vi "LMS Adaptive Filtering (V1.00).vi"(0 "Time Data":refnum<class "GSwFormDSP.lvclass">, 5 "error in (no error)":errorcluster, 7 "Application Name":string="AdvSigProc", 9 "State Queue":T3[](array[typedef])=["SC >>> Initialize"]) -> (19 "error out":errorcluster)   [LabVIEW 2020, in "AdvSigProc.lvclass"]
uses:
  AdvSigProc.lvclass
  API/Generic Utilities_class/utils/GenUtil State List.ctl
  API/GSwFormDSP_class/GSwFormDSP.lvclass
  protected/LMS Input Parameters.ctl
  <vilib>/Utility/sysdir.llb/System Directory Type.ctl
  API/GSwFormDSP_class/functions/Attribute Options.ctl
  SPWB_class/Controls/Analysis Type.ctl
  C:/Users/fcharett/docsWork/coding/20openSourceSPWB/API/Generic Utilities_class/Generic Utilities.lvclass
  <vilib>/Platform/browser.llb/Open URL in Default Browser (path).vi
  <vilib>/addons/_AddQ/G#Object/G#Object.lvclass
  API/Generic Utilities_class/Generic Utilities.lvclass
  File IO/TDMS_class/TDMS.lvclass
  SPWB_class/SPWB.lvclass
panel:
  in  "Task":T1(tab)
  in  "Noisy Signal (X +n)":u16(ring) items=["MidSunvisor Array Center", "Voice Signal"]
  in  "Reference Signal (X)":u16(ring) items=["MidSunvisor Array Center", "Voice Signal"]
  in  "Input Parameters":T2={"Type"=enum."Normalized LMS", "Filter Class"=enum."Noise Cancelling (BGN Ref)", "Filter Length"=256, "µ Parameters"={"Type"=enum."User Input", "step size"=1.0}, "Iterations"={"Current"=1, "Maximum"=1000}} {"µ Parameters"."step size" scale=1e-08..1.0}
  in  "LMS Start/Stop":bool
  in  "TDP LMS Results":bool
  out "Filter Coefs":dbl[](graph)
  in  "Filtered Signals":waveform(dbl)[](graph)
  out "Iterations.Current":i32
  in  "Open TDMS":bool
  in  "Time Signal":waveform(dbl)[](graph)
  out "Current File":path
  in  "AppData Folder":bool
  out "State History":string[](array[string])
  out "State Index":i32
  out "Exec Time":dbl
  in  "TimeOut":i32=-1 caption="msec"
  in  "Exit":bool
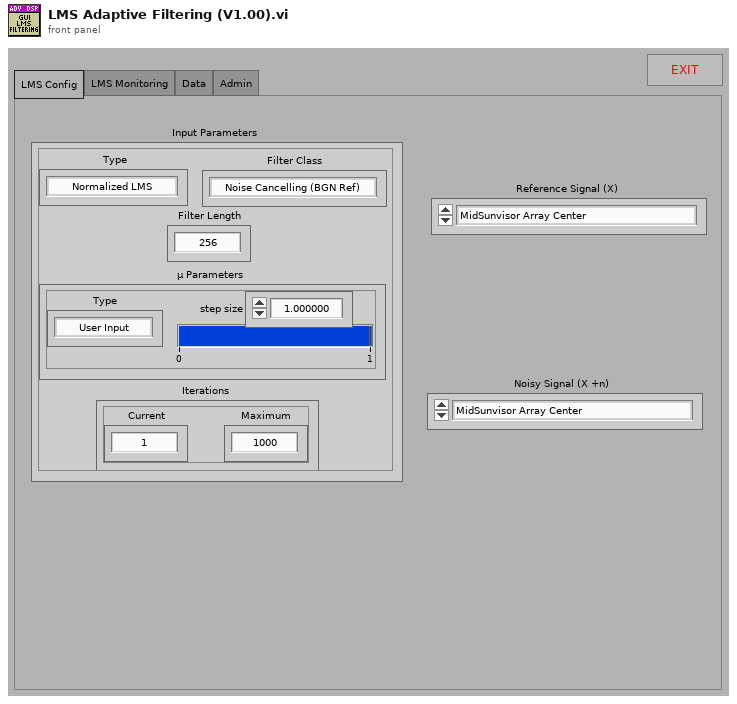
[diagram p1: front panel]
types:
  T1 = enum32{"LMS Config", "LMS Monitoring", "Data", "Admin"}
  T2 = typedef "AdvSigProc.lvclass/LMS Input Parameters.ctl" = cluster{"Type":enum16{"Normalized LMS", "LMS", "FIR Sign LMS", "FIR Fast Block LMS", "RLS", "QR - RLS"}, "Filter Class":enum16{"Noise Cancelling (BGN Ref)", "Noise Cancelling (Speech Ref)"}, "Filter Length":i32, "µ Parameters":cluster{"Type":enum16{"User Input", "Auto µ"}, "step size":dbl}, "Iterations":cluster{"Current":i32, "Maximum":i32}}
  T3 = typedef "Generic Utilities.lvclass/GenUtil State List.ctl" = string
  T4 = typedef "SPWB.lvclass/Analysis Type.ctl" = enum16{"Time Data Processing", "FFT Analysis", "Time Frequency Analysis", "Transfer Functions"}
  T5 = typedef "GSwFormDSP.lvclass/Attribute Options.ctl" = enum16{"Append to Attribute using \"( )\"", "Replace Attribute Value"}
  T6 = enum32{"Invalid", "Standard", "Closed", "Hidden", "Minimized", "Maximized"}
  T7 = typedef "System Directory Type.ctl" = i32
  T8 = cluster{"Window Name Index":string, "wForm Ref":refnum<class "GSwFormDSP.lvclass">}[]
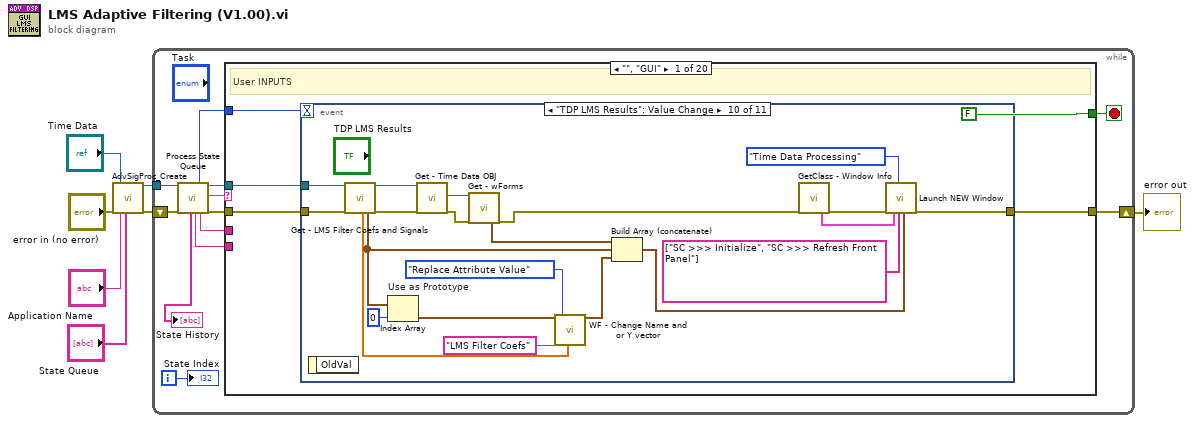
[diagram p0: block diagram]
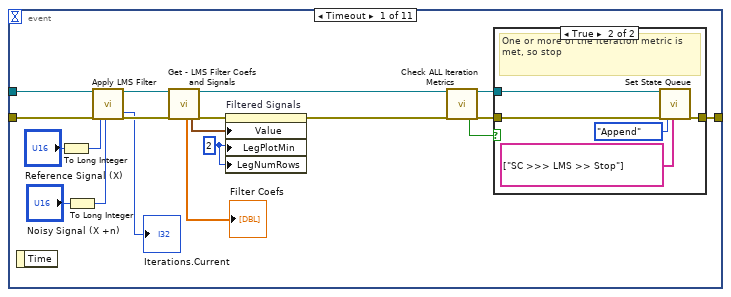
[diagram p2: hidden frame]
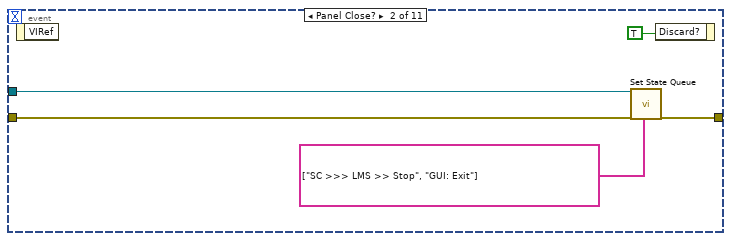
[diagram p4: hidden frame]
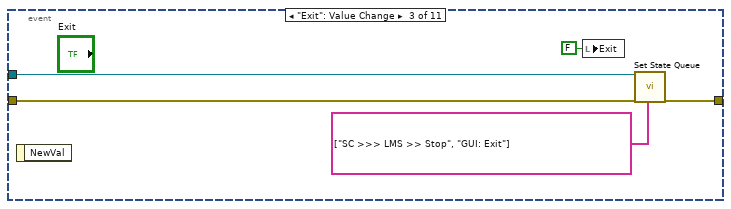
[diagram p5: hidden frame]
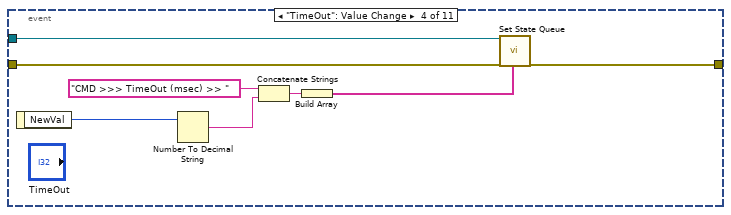
[diagram p6: hidden frame]
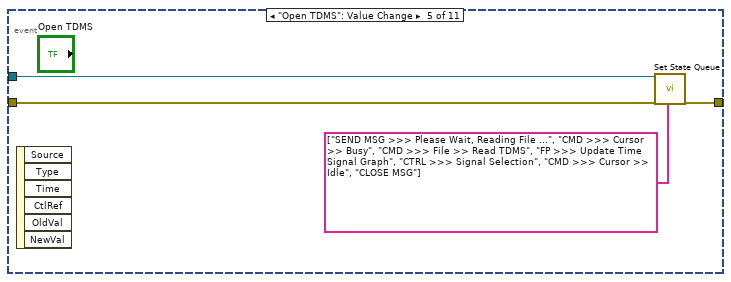
[diagram p7: hidden frame]
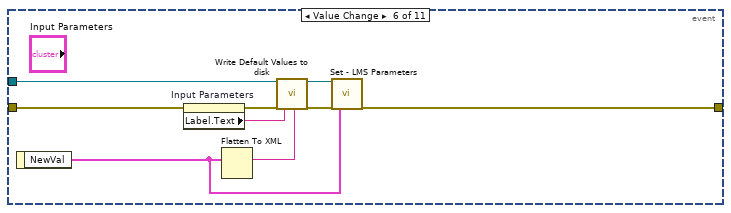
[diagram p8: hidden frame]
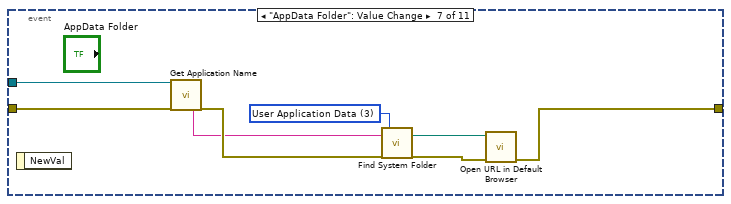
[diagram p9: hidden frame]
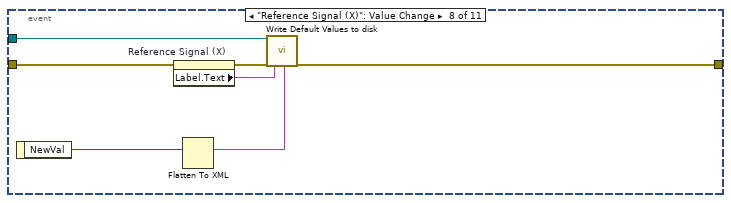
[diagram p10: hidden frame]
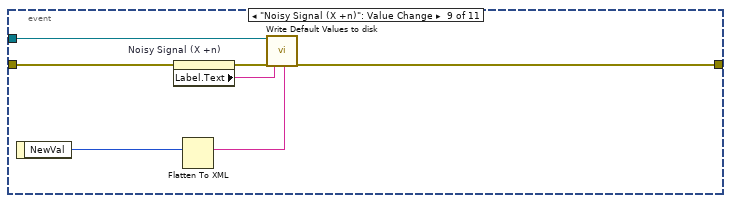
[diagram p11: hidden frame]
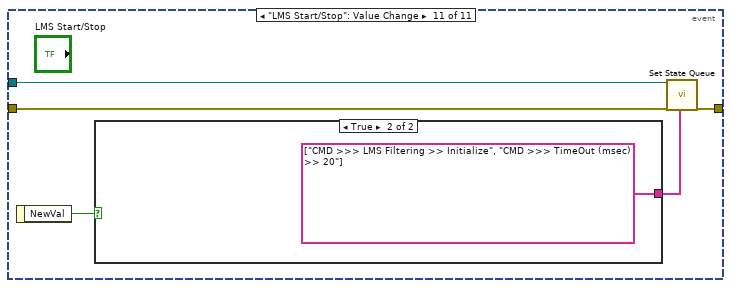
[diagram p12: hidden frame]
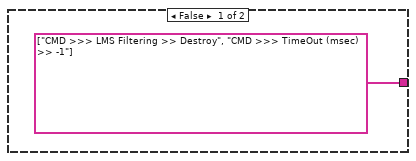
[diagram p13: hidden frame]
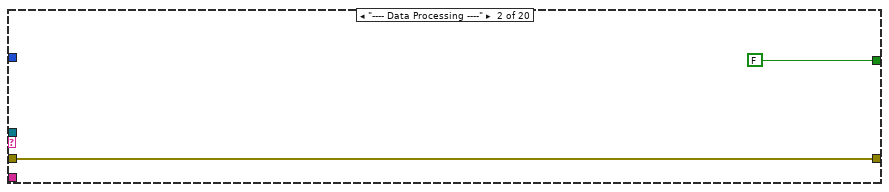
[diagram p14: hidden frame]
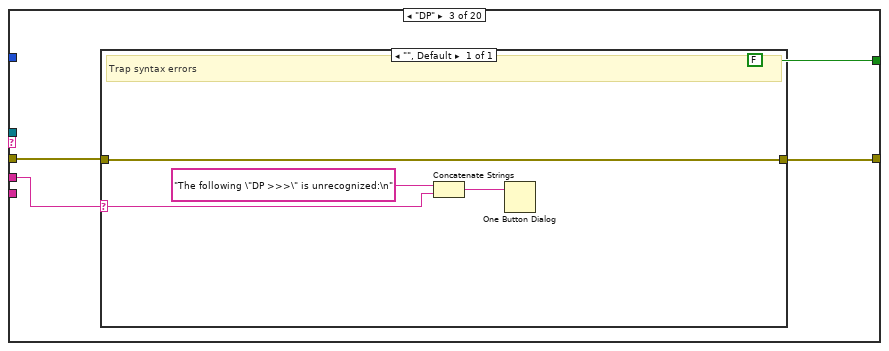
[diagram p15: hidden frame]
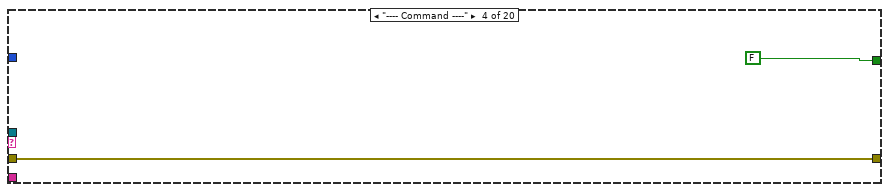
[diagram p16: hidden frame]
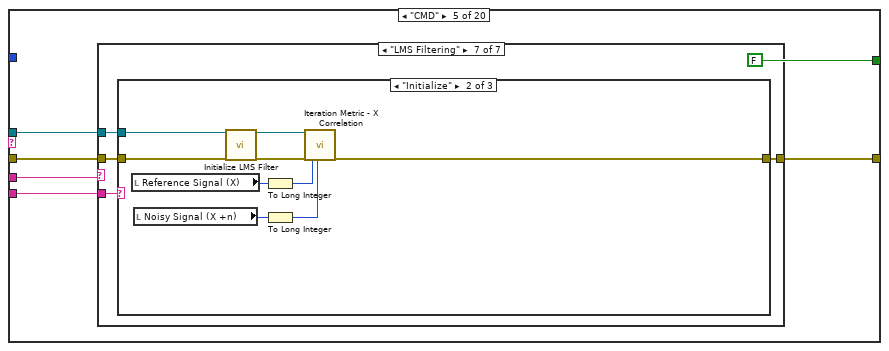
[diagram p17: hidden frame]
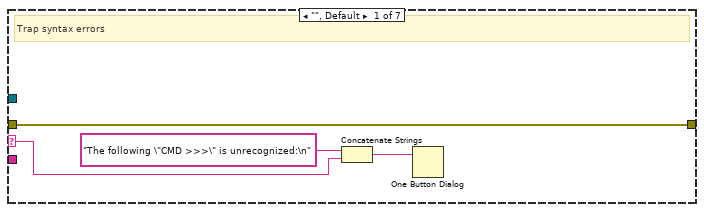
[diagram p18: hidden frame]
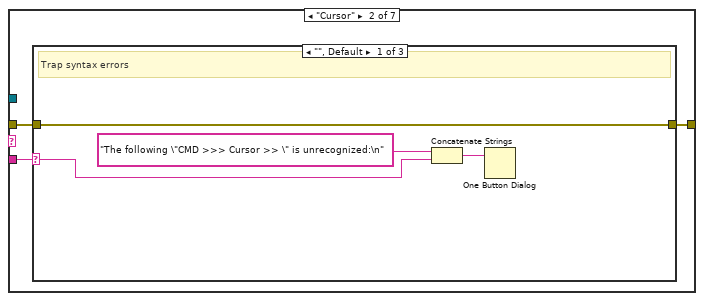
[diagram p19: hidden frame]
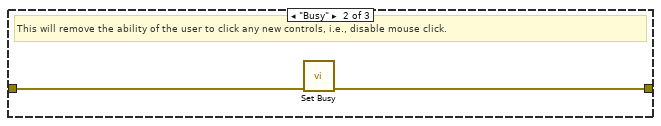
[diagram p20: hidden frame]
diagram:
  n1 = call "AdvSigProc_Create.vi"("error in (no error)"="error in (no error)", "Time Data"="Time Data", "Application Name"="Application Name", "State Queue"="State Queue") -> ("reference out"=w7:refnum<class "AdvSigProc.lvclass">, "error out"=w6:errorcluster)  [unwired: 14 in]
  n2 = while {
    shift-right: [w11] -> w2
    shift-left: w6 -> [w16]
    tunnel: w7 -> [w17]
    i -> [w18]
    stop <- w19 stop-if-true
    n3 = call "Process State Queue.vi"("reference in"=w17, "error in (no error)"=w16) -> ("State History"=→"State History":string[], "Additional Options"=w8:string, "Timeout"=w15:i32, "State Option"=w10:string, "reference out"=w14:refnum<class "AdvSigProc.lvclass">, "Current State"=w13:string, "error out"=w12:errorcluster)  [unwired: 10 in, 1 out]
    n4 = case shown="\"\", \"GUI\"" w13 {
      selector: w13 -> [_ _ _ _ _ _ _ _ _ _ _ _ _ _ _ _ w485 _ _ _]
      tunnel: w14 -> [w22 _ _ _ w143 _ w238 _ w257 w371 _ w413 w439 w474 w478 _ _ _ _ w495]
      tunnel: [FALSE FALSE FALSE FALSE FALSE FALSE FALSE FALSE FALSE FALSE FALSE FALSE TRUE FALSE FALSE FALSE FALSE FALSE FALSE TRUE] -> w19
      tunnel: w15 -> [w23 _ _ _ _ _ _ _ _ _ _ _ _ _ _ _ _ _ _ _]
      tunnel: w10 -> [_ _ w135 _ w147 _ w234 _ w258 w368 _ _ _ w471 _ _ _ _ _ _]
      tunnel: w12 -> [w21 w131 w134 w141 w145 w230 w237 w252 w255 w370 w399 w411 w436 w473 w479 w481 w483 w488 w491 w494]
      tunnel: [w20 w131 w133 w141 w146 w230 w236 w252 w256 w369 w399 w401 w435 w472 w477 w481 w483 errorcluster {"status"=FALSE, "code"=0, "source"=""} ("error out") w491 w493] -> w11
      tunnel: w8 -> [_ _ _ _ w144 _ w232 _ w254 _ _ _ _ _ _ _ _ _ _ _]
      frame "", "GUI" {
        # "User INPUTS"
        n5 = event shown="[9] \"TDP LMS Results\": Value Change" {
          selector: _ -> [_ _ _ _ _ _ _ _ _ _ _]
          dyn-events: _ -> [_ _ _ _ _ _ _ _ _ _ _]
          timeout: w23 -> [_ _ _ _ _ _ _ _ _ _ _]
          tunnel: w22 -> [w42 w53 w58 w63 w70 w80 w87 w92 w99 w121 w127]
          tunnel: w21 -> [w43 w52 w56 w62 w69 w77 w86 w93 w100 w120 w126]
          tunnel: [w30 w51 w57 w61 w71 w73 w81 w89 w96 w104 w125] -> w20
          event Timeout {
            w33 = u32 2
            n6 = event-data() -> ()  [unwired: 1 in, 1 out]
            n7 = To Long Integer(number="Reference Signal (X)") -> (32bit integer=w38:i32)
            n8 = To Long Integer(number="Noisy Signal (X +n)") -> (32bit integer=w39:i32)
            n9 = call "Apply LMS Filter.vi"("reference in"=w42, "error in (no error)"=w43, "Reference Signal"=w38, "Response Signal"=w39) -> ("Iterations.Current"=→"Iterations.Current":i32, "reference out"=w37:refnum<class "AdvSigProc.lvclass">, "error out"=w36:errorcluster)  [unwired: 13 in]
            n10 = call "Get - LMS Filter Coefs and Signals.vi"("reference in"=w37, "error in (no error)"=w36) -> ("Filter Coefs"=→"Filter Coefs":dbl[], "LMS Filtered Signals"=w34:waveform(dbl)[], "reference out"=w29:refnum<class "AdvSigProc.lvclass">, "error out"=w35:errorcluster)  [unwired: 14 in]
            n11 = property on="Filtered Signals" class="WFGraph (strict)"(error in=w35, "Value"=w34, "LegPlotMin"=w33, "LegNumRows"=w33) -> (error out=w27:errorcluster)  [unwired: 1 in, 1 out]
            n12 = call "Check ALL Iteration Metrics.vi"("reference in"=w29, "error in (no error)"=w27) -> ("Stop Iteration"=w25:bool, "reference out"=w28:refnum<class "AdvSigProc.lvclass">, "error out"=w26:errorcluster)  [unwired: 15 in]
            n13 = case shown="True" w25 {
              tunnel: w26 -> [w44 w48]
              tunnel: w28 -> [_ w47]
              tunnel: [w44 w46] -> w30
              frame False {
                # "Go to the next iteration!"
              }
              frame True {
                # "One or more of the iteration metric is met, so stop"
                n14 = call "Set State Queue.vi"("reference in"=w47, "error in (no error)"=w48, "State Queue Options"=enum16{"Replace", "Append", "Prepend"}."Append", "State Queue"=string[] ["SC >>> LMS >> Stop"]) -> ("error out"=w46:errorcluster)  [unwired: 14 in, 1 out]
              }
            }
          }
          event Panel Close? {
            n15 = event-data() -> ()  [unwired: 1 in, 1 out]
            n16 = call "Set State Queue.vi"("reference in"=w53, "error in (no error)"=w52, "State Queue"=string[] ["SC >>> LMS >> Stop", "GUI: Exit"]) -> ("error out"=w51:errorcluster)  [unwired: 15 in, 1 out]
            n17 = event-data("Discard?"=TRUE) -> ()  [unwired: 1 in, 1 out]
          }
          event "Exit": Value Change {
            n18 = event-data() -> ()  [unwired: 1 in, 1 out]
            n19 = local write "Exit"(FALSE ("Exit")) -> ()
            n20 = call "Set State Queue.vi"("reference in"=w58, "error in (no error)"=w56, "State Queue"=string[] ["SC >>> LMS >> Stop", "GUI: Exit"]) -> ("error out"=w57:errorcluster)  [unwired: 15 in, 1 out]
          }
          event "TimeOut": Value Change {
            n21 = event-data() -> ("NewVal"=w60:i32)  [unwired: 1 in]
            n22 = Number To Decimal String(number=w60) -> (decimal integer string=w65:string)  [unwired: 1 in]
            n23 = Concatenate Strings("CMD >>> TimeOut (msec) >> " ("String"), w65) -> (w66:string)
            n24 = Build Array(w66) -> (w67:string[])
            n25 = call "Set State Queue.vi"("reference in"=w63, "error in (no error)"=w62, "State Queue"=w67) -> ("error out"=w61:errorcluster)  [unwired: 15 in, 1 out]
          }
          event "Open TDMS": Value Change {
            n26 = event-data() -> ()  [unwired: 1 in, 6 out]
            n27 = call "Set State Queue.vi"("reference in"=w70, "error in (no error)"=w69, "State Queue"=string[] ["SEND MSG >>> Please Wait, Reading File ...", "CMD >>> Cursor >> Busy", "CMD >>> File >> Read TDMS", "FP >>> Update Time Signal Graph", "CTRL >>> Signal Selection", "CMD >>> Cursor >> Idle", "CLOSE MSG"]) -> ("error out"=w71:errorcluster)  [unwired: 15 in, 1 out]
          }
          event Value Change {
            n28 = event-data() -> ("NewVal"=w72:T2)  [unwired: 1 in]
            n29 = property on="Input Parameters" class="Clust (strict)"(error in=w77) -> (error out=w76:errorcluster, "Label.Text"=w79:string)  [unwired: 1 in, 1 out]
            n30 = Flatten To XML(6:w72) -> (2:w78:string)
            n31 = call-dynamic "Write Default Values to disk.vi"("reference in"=w80, "error in (no error)"=w76, "Control Label"=w79, "Value (XML String)"=w78) -> ("reference out"=w74:refnum<class "AdvSigProc.lvclass">, "error out"=w75:errorcluster)  [unwired: 14 in]
            n32 = call "Set - LMS Parameters.vi"("reference in"=w74, "error in (no error)"=w75, "Input Parameters"=w72) -> ("error out"=w73:errorcluster)  [unwired: 15 in, 1 out]
          }
          event "AppData Folder": Value Change {
            w88 = T7 3 items=["User Home"=0, "User Desktop"=1, "User Documents"=2, "User Application Data"=3, "User Preferences"=4, "User Temporary"=5, "Public Documents"=6, "Public Application Data"=7, "Public Preferences"=8, "Public Cache"=13, "System Core Libraries"=9, "System Installed Libraries"=10, "Application Files"=11, "Boot Volume Root"=12] ("system directory type")
            n33 = event-data() -> ()  [unwired: 1 in, 1 out]
            n34 = call "Get Application Name.vi"("reference in"=w87, "error in (no error)"=w86) -> ("Application Name"=w84:string, "error out"=w85:errorcluster)  [unwired: 15 in, 1 out]
            n35 = call "Find System Folder.vi"("Application Name"=w84, "error in (no error)"=w85, "system directory type"=w88) -> ("System Folder"=w83:path, "error out"=w82:errorcluster)  [unwired: 15 in]
            n36 = call-poly <vilib>:"Open URL in Default Browser.vi"("error in (no error)"=w82, "path"=w83) -> ("error out"=w81:errorcluster)  [unwired: 4 in, 1 out]
          }
          event "Reference Signal (X)": Value Change {
            n37 = event-data() -> ("NewVal"=w91:u16)  [unwired: 1 in]
            n38 = property on="Reference Signal (X)" class="Ring (strict)"(error in=w93) -> (error out=w94:errorcluster, "Label.Text"=w95:string)  [unwired: 1 in, 1 out]
            n39 = Flatten To XML(6:w91) -> (2:w90:string)
            n40 = call-dynamic "Write Default Values to disk.vi"("reference in"=w92, "error in (no error)"=w94, "Control Label"=w95, "Value (XML String)"=w90) -> ("error out"=w89:errorcluster)  [unwired: 14 in, 1 out]
          }
          event "Noisy Signal (X +n)": Value Change {
            n41 = event-data() -> ("NewVal"=w98:u16)  [unwired: 1 in]
            n42 = property on="Noisy Signal (X +n)" class="Ring (strict)"(error in=w100) -> (error out=w101:errorcluster, "Label.Text"=w102:string)  [unwired: 1 in, 1 out]
            n43 = Flatten To XML(6:w98) -> (2:w97:string)
            n44 = call-dynamic "Write Default Values to disk.vi"("reference in"=w99, "error in (no error)"=w101, "Control Label"=w102, "Value (XML String)"=w97) -> ("error out"=w96:errorcluster)  [unwired: 14 in, 1 out]
          }
          event "TDP LMS Results": Value Change {
            n45 = event-data() -> ()  [unwired: 1 in, 1 out]
            n46 = call "Get - LMS Filter Coefs and Signals.vi"("reference in"=w121, "error in (no error)"=w120) -> ("Filter Coefs"=w116:dbl[], "LMS Filtered Signals"=w111:waveform(dbl)[], "reference out"=w119:refnum<class "AdvSigProc.lvclass">, "error out"=w118:errorcluster)  [unwired: 14 in]
            n47 = Index Array "Use as Prototype"(array=w111, index=0) -> (element=w113:waveform(dbl))
            n48 = call "Get - Time Data OBJ.vi"("reference in"=w119, "error in (no error)"=w118) -> ("GSwFormDSP"=w123:refnum<class "GSwFormDSP.lvclass">, "error out"=w122:errorcluster)  [unwired: 14 in, 2 out]
            n49 = call-dynamic "Get - wForms.vi"("reference in"=w123, "error in (no error)"=w122) -> ("wForms"=w110:waveform(dbl)[], "error out"=w106:errorcluster)  [unwired: 14 in, 2 out]
            n50 = call "WF - Change Name and or Y vector.vi"("wForm IN"=w113, "Attribute Option"=Attribute_Options."Replace Attribute Value", "SigName Update"="LMS Filter Coefs", "New Y Data"=w116) -> ("wForm OUT"=w112:waveform(dbl))  [unwired: 14 in, 1 out]
            n51 = Build Array (concatenate)(w110, w111, w112) -> (w105:waveform(dbl)[])
            n52 = call "GetClass - Window Info.vi"("error in (no error)"=w106) -> ("Window Info"=w109:T8, "error out"=w108:errorcluster)  [unwired: 17 in]
            n53 = call "Launch NEW Window.vi"("error in (no error)"=w108, "Window Info"=w109, "Window Type"=Analysis_Type."Time Data Processing", "State Queue"=string[] ["SC >>> Initialize", "SC >>> Refresh Front Panel"], "wForms"=w105) -> ("error OUT"=w104:errorcluster)  [unwired: 14 in]
          }
          event "LMS Start/Stop": Value Change {
            n54 = event-data() -> ("NewVal"=w124:bool)  [unwired: 1 in]
            n55 = case shown="True" w124 {
              tunnel: [string[] ["CMD >>> LMS Filtering >> Destroy", "CMD >>> TimeOut (msec) >> -1"] ("State Queue") string[] ["CMD >>> LMS Filtering >> Initialize", "CMD >>> TimeOut (msec) >> 20"] ("State Queue")] -> w128
              frame False {
              }
              frame True {
              }
            }
            n56 = call "Set State Queue.vi"("reference in"=w127, "error in (no error)"=w126, "State Queue"=w128) -> ("error out"=w125:errorcluster)  [unwired: 15 in, 1 out]
          }
        }
      }
      frame "---- Data Processing ----" {
      }
      frame "DP" {
        n57 = case shown="\"\", Default" w135 {
          selector: w135 -> [w138]
          tunnel: [w137] -> w133
          tunnel: w134 -> [w137]
          frame "", Default {
            # "Trap syntax errors"
            n58 = Concatenate Strings("The following \"DP >>>\" is unrecognized:\n", w138) -> (w139:string)
            n59 = One Button Dialog(message=w139) -> ()  [unwired: 1 in, 1 out]
          }
        }
      }
      frame "---- Command ----" {
      }
      frame "CMD" {
        n60 = case shown="\"LMS Filtering\"" w147 {
          selector: w147 -> [w150 _ _ _ _ _ _]
          tunnel: [w149 w154 w166 w185 w187 w194 w212] -> w146
          tunnel: w145 -> [w149 w153 w165 w185 w188 w193 w211]
          tunnel: w144 -> [_ w155 w167 w182 w190 w195 w213]
          tunnel: w143 -> [_ _ w164 _ w189 w192 w210]
          frame "", Default {
            # "Trap syntax errors"
            n61 = Concatenate Strings("The following \"CMD >>>\" is unrecognized:\n", w150) -> (w151:string)
            n62 = One Button Dialog(message=w151) -> ()  [unwired: 1 in, 1 out]
          }
          frame "Cursor" {
            n63 = case shown="\"\", Default" w155 {
              selector: w155 -> [w157 _ _]
              tunnel: [w156 w160 w162] -> w154
              tunnel: w153 -> [w156 w161 w163]
              frame "", Default {
                # "Trap syntax errors"
                n64 = Concatenate Strings("The following \"CMD >>> Cursor >> \" is unrecognized:\n", w157) -> (w158:string)
                n65 = One Button Dialog(message=w158) -> ()  [unwired: 1 in, 1 out]
              }
              frame "Busy" {
                # "This will remove the ability of the user to click any new controls, i.e., disable mouse click."
                n66 = call <vilib>:"Set Busy.vi"("error in (no error)"=w161) -> ("error out"=w160:errorcluster)  [unwired: 9 in, 1 out]
              }
              frame "Idle" {
                # "Re-enables mouse click"
                n67 = call <vilib>:"Unset Busy.vi"("error in (no error)"=w163) -> ("error out"=w162:errorcluster)  [unwired: 10 in]
              }
            }
          }
          frame "Timer" {
            # "Can be use to time the execution or delays in processing or acquisition."
            n68 = case shown="\"\", Default" w167 {
              selector: w167 -> [w169 _ _]
              tunnel: [w168 w173 w178] -> w166
              tunnel: w165 -> [w168 w174 w179]
              tunnel: w164 -> [_ w175 w180]
              frame "", Default {
                # "Trap syntax errors"
                n69 = Concatenate Strings("The following \"CMD >>> Timer >> \" is unrecognized:\n", w169) -> (w170:string)
                n70 = One Button Dialog(message=w170) -> ()  [unwired: 1 in, 1 out]
              }
              frame "Start" {
                n71 = Get Date/Time In Seconds() -> (seconds since 1Jan1904=w172:timestamp)
                n72 = call "Set Timer Start.vi"("reference in"=w175, "error in (no error)"=w174, "Timer Start"=w172) -> ("error out"=w173:errorcluster)  [unwired: 15 in, 1 out]
              }
              frame "Stop" {
                n73 = call "Get Timer Start.vi"("reference in"=w180, "error in (no error)"=w179) -> ("Timer Start"=w177:timestamp, "error out"=w178:errorcluster)  [unwired: 15 in, 1 out]
                n74 = Get Date/Time In Seconds() -> (seconds since 1Jan1904=w181:timestamp)
                n75 = Subtract(x=w181, y=w177) -> (x-y=→"Exec Time":dbl)
              }
            }
          }
          frame "Wait (ms)" {
            # "Forces a time out"
            n76 = Decimal String To Number(string=w182, default (0L)=u32 0 ("default (0 I32)")) -> (number=w183:u32)  [unwired: 1 in, 1 out]
            n77 = Wait (ms)(milliseconds to wait=w183) -> ()  [unwired: 1 out]
          }
          frame "TimeOut (msec)" {
            # "Setup the default loop time out"
            n78 = Decimal String To Number(string=w190, default (0L)=0 ("default (0 I32)")) -> (number=w186:i32)  [unwired: 1 in, 1 out]
            n79 = call "Set State TimeOut.vi"("reference in"=w189, "error in (no error)"=w188, "TimeOut (msec)"=w186) -> ("error out"=w187:errorcluster)  [unwired: 15 in, 1 out]
            n80 = local write "TimeOut"(w186) -> ()
          }
          frame "File" {
            n81 = case shown="\"Read TDMS\"" w195 {
              selector: w195 -> [w197 _]
              tunnel: [w196 w200] -> w194
              tunnel: w193 -> [w196 w208]
              tunnel: w192 -> [_ w209]
              frame "", Default {
                n82 = Concatenate Strings("The following \"CMD >>> File >>\" is unrecognized:\n", w197) -> (w198:string)
                n83 = One Button Dialog(message=w198) -> ()  [unwired: 1 in, 1 out]
              }
              frame "Read TDMS" {
                n84 = call "Get Application Name.vi"("reference in"=w209, "error in (no error)"=w208) -> ("Application Name"=w203:string, "reference out"=w207:refnum<class "AdvSigProc.lvclass">, "error out"=w206:errorcluster)  [unwired: 15 in]
                n85 = call "Get - Time Data OBJ.vi"("reference in"=w207, "error in (no error)"=w206) -> ("GSwFormDSP"=w205:refnum<class "GSwFormDSP.lvclass">, "error out"=w204:errorcluster)  [unwired: 14 in, 2 out]
                n86 = call "GUI - TDMS (V2.00).vi"("Time Data IN"=w205, "error in (no error)"=w204, "Application Name"=w203, "State Queue"=string[] ["CMD: Prompt For READ Path", "CMD: Read File", "Quit"]) -> ("Loaded File"=→"Current File":path, "error out"=w200:errorcluster)  [unwired: 13 in, 1 out]
              }
            }
          }
          frame "LMS Filtering" {
            n87 = case shown="\"Initialize\"" w213 {
              selector: w213 -> [w215 _ _]
              tunnel: [w214 w218 w227] -> w212
              tunnel: w211 -> [w214 w225 w228]
              tunnel: w210 -> [_ w226 w229]
              frame "", Default {
                n88 = Concatenate Strings("The following \"CMD >>> LMS Filtering >>\" is unrecognized:\n", w215) -> (w216:string)
                n89 = One Button Dialog(message=w216) -> ()  [unwired: 1 in, 1 out]
              }
              frame "Initialize" {
                n90 = local read "Reference Signal (X)"() -> (w222:u16)
                n91 = local read "Noisy Signal (X +n)"() -> (w220:u16)
                n92 = call "Initialize LMS Filter.vi"("reference in"=w226, "error in (no error)"=w225) -> ("reference out"=w223:refnum<class "AdvSigProc.lvclass">, "error out"=w224:errorcluster)  [unwired: 16 in]
                n93 = To Long Integer(number=w222) -> (32bit integer=w221:i32)
                n94 = To Long Integer(number=w220) -> (32bit integer=w219:i32)
                n95 = call "Iteration Metric - X Correlation.vi"("reference in"=w223, "error in (no error)"=w224, "Reference Signal"=w221, "Response Signal"=w219) -> ("error out"=w218:errorcluster)  [unwired: 14 in, 1 out]
              }
              frame "Destroy" {
                n96 = call "Destroy LMS Filter.vi"("reference in"=w229, "error in (no error)"=w228) -> ("error out"=w227:errorcluster)  [unwired: 16 in, 1 out]
              }
            }
          }
        }
      }
      frame "---- Scripts ----" {
      }
      frame "SC" {
        n97 = case shown="\"LMS\"" w234 {
          selector: w234 -> [w241 _ _]
          tunnel: [string[] [] ("State Queue OUT") string[] ["GUI: Initialize Ref", "CTRL >>> Task Tab", "CTRL >>> LMS Parameters", "FP >>> Open"] ("State Queue OUT") w245] -> w235
          tunnel: w232 -> [_ _ w246]
          frame "False", Default {
            n98 = Concatenate Strings("The following \"Script\" is unrecognized:\n", w241) -> (w242:string)
            n99 = One Button Dialog(message=w242) -> ()  [unwired: 1 in, 1 out]
          }
          frame "Initialize" {
          }
          frame "LMS" {
            n100 = case shown="\"Stop\"" w246 {
              selector: w246 -> [w248 _]
              tunnel: [string[] [] ("State Queue OUT") string[] ["CMD >>> TimeOut (msec) >> -1", "CMD >>> LMS Filtering >> Destroy", "CTRL >>> LMS >> Stop"] ("State Queue OUT")] -> w245
              frame "", Default {
                n101 = Concatenate Strings("The following \"SC >>> LMS\" is unrecognized:\n", w248) -> (w249:string)
                n102 = One Button Dialog(message=w249) -> ()  [unwired: 1 in, 1 out]
              }
              frame "Stop" {
              }
            }
          }
        }
        n103 = call "Set State Queue.vi"("reference in"=w238, "error in (no error)"=w237, "State Queue Options"=enum16{"Replace", "Append", "Prepend"}."Prepend", "State Queue"=w235) -> ("error out"=w236:errorcluster)  [unwired: 14 in, 1 out]
      }
      frame "---- Front Panel Mgmt ----" {
      }
      frame "CTRL" {
        n104 = case shown="\"Signal Selection\"" w258 {
          selector: w258 -> [w262 _ _ _ _]
          tunnel: w257 -> [_ w267 w294 w330 _]
          tunnel: [w260 w265 w287 w305 w360] -> w256
          tunnel: w255 -> [w260 w266 w292 w329 w359]
          tunnel: w254 -> [_ _ _ _ w361]
          frame "unknown", Default {
            n105 = Concatenate Strings("The following control name is unrecognized:\n", w262) -> (w261:string)
            n106 = One Button Dialog(message=w261) -> ()  [unwired: 1 in, 1 out]
          }
          frame "Task Tab" {
            n107 = disable-structure shown="Enabled" {
              disable-tunnel: [w276 0] -> w268
              disable-tunnel: w267 -> [w274 _]
              disable-tunnel: w266 -> [w272 w284]
              disable-tunnel: [w269 w284] -> w264
              frame Disabled {
                n108 = property on="Task" class="TabCtl (strict)"(error in=w272) -> (error out=w273:errorcluster, "Label.Text"=w271:string, "Value"=w275:T1)  [unwired: 1 in, 1 out]
                n109 = call-dynamic "Read Default Values from Disk.vi"("reference in"=w274, "error in (no error)"=w273, "Control Label"=w271) -> ("Value (XML String)"=w270:string, "error out"=w269:errorcluster)  [unwired: 14 in, 1 out]
                n110 = case shown="\"anything\", Default" w270 {
                  selector: w270 -> [w281 _]
                  tunnel: [w277 w282] -> w276
                  tunnel: w275 -> [w279 w282]
                  frame "anything", Default {
                    # "Decode XML"
                    n111 = Unflatten From XML(xml string=w281, type=w279) -> (value=w278:T1, error out=w280:errorcluster)  [unwired: 1 in]
                    n112 = Select(t=w279, s=w280, f=w278) -> (s? t:f=w277:T1)
                  }
                  frame "" {
                    # "NO File / Error"
                  }
                }
              }
              frame Enabled {
              }
            }
            n113 = property on="Task" class="TabCtl (strict)"(error in=w264, "Value"=w268) -> (error out=w265:errorcluster)  [unwired: 1 in, 1 out]
          }
          frame "LMS Parameters" {
            n114 = property on="Input Parameters" class="Clust (strict)"(error in=w292) -> (error out=w293:errorcluster, "Label.Text"=w291:string, "Value"=w295:T2)  [unwired: 1 in, 1 out]
            n115 = call-dynamic "Read Default Values from Disk.vi"("reference in"=w294, "error in (no error)"=w293, "Control Label"=w291) -> ("Value (XML String)"=w290:string, "reference out"=w286:refnum<class "AdvSigProc.lvclass">, "error out"=w289:errorcluster)  [unwired: 14 in]
            n116 = case shown="\"anything\", Default" w290 {
              selector: w290 -> [w300 _]
              tunnel: [w296 w301] -> w285
              tunnel: w295 -> [w298 w301]
              frame "anything", Default {
                # "Decode XML"
                n117 = Unflatten From XML(xml string=w300, type=w298) -> (value=w297:T2, error out=w299:errorcluster)  [unwired: 1 in]
                n118 = Select(t=w298, s=w299, f=w297) -> (s? t:f=w296:T2)
              }
              frame "" {
                # "NO File / Error"
              }
            }
            n119 = property on="Input Parameters" class="Clust (strict)"(error in=w289, "Value"=w285) -> (error out=w288:errorcluster)  [unwired: 1 in, 1 out]
            n120 = call "Set - LMS Parameters.vi"("reference in"=w286, "error in (no error)"=w288, "Input Parameters"=w285) -> ("error out"=w287:errorcluster)  [unwired: 15 in, 1 out]
          }
          frame "Signal Selection" {
            n121 = call "Get - Time Data OBJ.vi"("reference in"=w330, "error in (no error)"=w329) -> ("GSwFormDSP"=w328:refnum<class "GSwFormDSP.lvclass">, "error out"=w327:errorcluster)  [unwired: 14 in, 2 out]
            n122 = call-dynamic "Get - Names and Units.vi"("reference in"=w328, "error in (no error)"=w327) -> ("Signal Names"=w302:string[], "reference out"=w323:refnum<class "GSwFormDSP.lvclass">, "error out"=w326:errorcluster)  [unwired: 13 in, 2 out]
            n123 = property on="Reference Signal (X)" class="Ring (strict)"(error in=w326, "Strings []"=w302) -> (error out=w324:errorcluster, "Label.Text"=w322:string, "Value"=w321:u16)  [unwired: 1 in, 1 out]
            n124 = Array Size(array=w302) -> (size(s)=w304:i32)
            n125 = disable-structure shown="Enabled" {
              disable-tunnel: [w343 w344] -> w325
              disable-tunnel: w324 -> [w342 w345]
              disable-tunnel: w323 -> [w341 w346]
              disable-tunnel: w322 -> [w340 w344]
              disable-tunnel: [w339 w345] -> w317
              disable-tunnel: [w338 w346] -> w303
              frame Disabled {
                n126 = call-dynamic "Read Default Values from Disk.vi"("reference in"=w341, "error in (no error)"=w342, "Control Label"=w340) -> ("Value (XML String)"=w343:string, "reference out"=w338:refnum<class "GSwFormDSP.lvclass">, "error out"=w339:errorcluster)  [unwired: 14 in]
              }
              frame Enabled {
              }
            }
            n127 = case shown="\"anything\", Default" w325 {
              selector: w325 -> [w357 _]
              tunnel: [w353 w358] -> w319
              tunnel: w321 -> [w355 w358]
              frame "anything", Default {
                # "Decode XML"
                n128 = Unflatten From XML(xml string=w357, type=w355) -> (value=w354:u16, error out=w356:errorcluster)  [unwired: 1 in]
                n129 = Select(t=w355, s=w356, f=w354) -> (s? t:f=w353:u16)
              }
              frame "" {
                # "NO File / Error"
              }
            }
            n130 = Less?(x=w319, y=w304) -> (x < y?=w320:bool)
            n131 = Select(t=w319, s=w320, f=u16 0) -> (s? t:f=w316:u16)
            n132 = property on="Reference Signal (X)" class="Ring (strict)"(error in=w317, "Value"=w316) -> (error out=w306:errorcluster)  [unwired: 1 in, 1 out]
            n133 = property on="Noisy Signal (X +n)" class="Ring (strict)"(error in=w306, "Strings []"=w302) -> (error out=w308:errorcluster, "Label.Text"=w309:string, "Value"=w310:u16)  [unwired: 1 in, 1 out]
            n134 = disable-structure shown="Enabled" {
              disable-tunnel: [w335 w337] -> w314
              disable-tunnel: w309 -> [w334 w336]
              disable-tunnel: w308 -> [w333 w337]
              disable-tunnel: [w332 w336] -> w307
              disable-tunnel: w303 -> [w331 _]
              frame Disabled {
                n135 = call-dynamic "Read Default Values from Disk.vi"("reference in"=w331, "error in (no error)"=w333, "Control Label"=w334) -> ("Value (XML String)"=w332:string, "error out"=w335:errorcluster)  [unwired: 14 in, 1 out]
              }
              frame Enabled {
              }
            }
            n136 = case shown="\"anything\", Default" w307 {
              selector: w307 -> [w351 _]
              tunnel: [w347 w352] -> w312
              tunnel: w310 -> [w349 w352]
              frame "anything", Default {
                # "Decode XML"
                n137 = Unflatten From XML(xml string=w351, type=w349) -> (value=w348:u16, error out=w350:errorcluster)  [unwired: 1 in]
                n138 = Select(t=w349, s=w350, f=w348) -> (s? t:f=w347:u16)
              }
              frame "" {
                # "NO File / Error"
              }
            }
            n139 = Less?(x=w312, y=w304) -> (x < y?=w311:bool)
            n140 = Select(t=w312, s=w311, f=u16 0) -> (s? t:f=w315:u16)
            n141 = property on="Noisy Signal (X +n)" class="Ring (strict)"(error in=w314, "Value"=w315) -> (error out=w305:errorcluster)  [unwired: 1 in, 1 out]
          }
          frame "LMS" {
            n142 = case shown="\"Stop\"" w361 {
              selector: w361 -> [w363 _]
              tunnel: [w362 w366] -> w360
              tunnel: w359 -> [w362 w366]
              frame "", Default {
                n143 = Concatenate Strings("The following \"CTRL >>> LMS >> \" name is unrecognized:\n", w363) -> (w364:string)
                n144 = One Button Dialog(message=w364) -> ()  [unwired: 1 in, 1 out]
              }
              frame "Stop" {
                n145 = local write "LMS Start/Stop"(FALSE ("LMS Start/Stop")) -> ()
              }
            }
          }
        }
      }
      frame "FP" {
        n146 = case shown="\"Update Time Signal Graph\"" w368 {
          selector: w368 -> [w373 _ _]
          tunnel: w371 -> [_ w381 w394]
          tunnel: w370 -> [w374 w380 w393]
          tunnel: [w374 w377 w392] -> w369
          frame "unknown", Default {
            n147 = Concatenate Strings("The following FP Command name is unrecognized:\n", w373) -> (w375:string)
            n148 = One Button Dialog(message=w375) -> ()  [unwired: 1 in, 1 out]
          }
          frame "Open" {
            n149 = call-dynamic "Get VI Ref.vi"("reference in"=w381, "error in (no error)"=w380) -> ("GUI VI Ref"=w378:refnum<vi>, "error out"=w379:errorcluster)  [unwired: 14 in, 2 out]
            n150 = property class="VI"(reference=w378, error in=w379) -> (reference out=w383:refnum<vi>, error out=w384:errorcluster, "Front Panel.Open"=w382:bool)
            n151 = case shown="False" w382 {
              tunnel: [w387 w390] -> w377
              tunnel: w384 -> [w386 w390]
              tunnel: w383 -> [w385 _]
              frame False {
                n152 = invoke class="VI" method="FP.Open"(reference=w385, error in=w386, "Activate"=TRUE, "State"=T6."Standard") -> (error out=w387:errorcluster)  [unwired: 1 in, 4 out]
              }
              frame True {
              }
            }
          }
          frame "Update Time Signal Graph" {
            n153 = call "Get - Time Data OBJ.vi"("reference in"=w394, "error in (no error)"=w393) -> ("GSwFormDSP"=w395:refnum<class "GSwFormDSP.lvclass">, "error out"=w396:errorcluster)  [unwired: 14 in, 2 out]
            n154 = call-dynamic "Get - wForms.vi"("reference in"=w395, "error in (no error)"=w396) -> ("Nb Signals"=w391:i32, "wForms"=w398:waveform(dbl)[], "error out"=w397:errorcluster)  [unwired: 14 in, 1 out]
            n155 = property on="Time Signal" class="WFGraph (strict)"(error in=w397, "Value"=w398, "LegPlotMin"=w391, "LegNumRows"=w391) -> (error out=w392:errorcluster)  [unwired: 1 in, 1 out]
          }
        }
      }
      frame "---- GUI Functions ----" {
      }
      frame "GUI: Initialize Ref" {
        n156 = call "Get - Time Data OBJ.vi"("reference in"=w413, "error in (no error)"=w411) -> ("New Time Data Obj?"=w408:bool, "reference out"=w414:refnum<class "AdvSigProc.lvclass">, "GSwFormDSP"=w409:refnum<class "GSwFormDSP.lvclass">, "error out"=w412:errorcluster)  [unwired: 14 in]
        n157 = control-ref of="GUI Reference"() -> (w418:refnum<vi>)
        n158 = call "Set VI Ref.vi"("reference in"=w414, "error in (no error)"=w412, "ReInit All to Default?"=w408, "GUI VI Ref"=w418) -> ("reference out"=w420:refnum<class "AdvSigProc.lvclass">, "error out"=w417:errorcluster)  [unwired: 14 in]
        n159 = call "Set Close Panel (Yes or No).vi"("reference in"=w420, "error in (no error)"=w417) -> ("reference out"=w419:refnum<class "AdvSigProc.lvclass">, "error out"=w416:errorcluster)  [unwired: 16 in]
        n160 = call "Set Message Window Ref.vi"("reference in"=w419, "error in (no error)"=w416) -> ("reference out"=w406:refnum<class "AdvSigProc.lvclass">, "error out"=w410:errorcluster)  [unwired: 16 in]
        n161 = case shown="True" w408 {
          tunnel: w409 -> [_ w427]
          tunnel: w410 -> [w422 w425]
          tunnel: "Time Signal" -> [_ w424]
          tunnel: [w422 w423] -> w407
          frame False {
          }
          frame True {
            n162 = call "Set - wForms.vi"("reference in"=w427, "error in (no error)"=w425, "Init wForms"=TRUE, "wForms"=w424) -> ("error out"=w423:errorcluster)  [unwired: 14 in, 1 out]
          }
        }
        n163 = call "Get - LMS Filtered Signals OBJ.vi"("reference in"=w406, "error in (no error)"=w407) -> ("GSwFormDSP"=w403:refnum<class "GSwFormDSP.lvclass">, "error out"=w404:errorcluster)  [unwired: 15 in, 1 out]
        n164 = call "Set - wForms.vi"("reference in"=w403, "error in (no error)"=w404, "Init wForms"=TRUE, "wForms"="Filtered Signals") -> ("error out"=w401:errorcluster)  [unwired: 14 in, 1 out]
      }
      frame "GUI: Exit" {
        n165 = call-dynamic "Get Message Window Ref.vi"("reference in"=w439, "error in (no error)"=w436) -> ("reference out"=w438:refnum<class "AdvSigProc.lvclass">, "Msg Win Ref"=w434:refnum<vi>, "error out"=w437:errorcluster)  [unwired: 15 in]
        n166 = call-dynamic "Get VI Ref.vi"("reference in"=w438, "error in (no error)"=w437) -> ("reference out"=w442:refnum<class "AdvSigProc.lvclass">, "GUI VI Ref"=w440:refnum<vi>, "error out"=w441:errorcluster)  [unwired: 14 in, 1 out]
        n167 = call-dynamic "Get Close Panel (Yes or No).vi"("reference in"=w442, "error in (no error)"=w441) -> ("Close Panel?"=w443:bool, "reference out"=w432:refnum<class "AdvSigProc.lvclass">, "error out"=w433:errorcluster)  [unwired: 15 in]
        n168 = call-dynamic "Get OBJ NOT RefNum.vi"("reference in"=w432, "error in (no error)"=w433) -> ("OBJ not a refnum?"=w431:bool, "reference out"=w430:refnum<class "AdvSigProc.lvclass">, "error out"=w429:errorcluster)  [unwired: 15 in]
        n169 = case shown="True" w431 {
          tunnel: [w448 w451] -> w428
          tunnel: w430 -> [_ w450]
          tunnel: w429 -> [w448 w449]
          frame False {
            # "The OBJ already exist, indicating this is a dialog box or sub-vi so do NOT destroy the original OBJ."
          }
          frame True {
            # "New OBJ was created, so it needs to be deleted."
            n170 = call-dynamic "Destroy.vi"("reference in"=w450, "error in (no error)"=w449) -> ("error out"=w452:errorcluster)  [unwired: 16 in, 1 out]
            n171 = disable-structure shown="Disabled" {
              disable-tunnel: w452 -> [w454 w455]
              disable-tunnel: [w453 w455] -> w451
              frame Disabled {
                # "Enable when NEEDED"
                n172 = call <vilib>:"GarbageCollector.vi"("error in (no error)"=w454) -> ("error out"=w453:errorcluster)  [unwired: 16 in, 2 out]
              }
              frame Enabled {
              }
            }
          }
        }
        n173 = Close Reference(reference=w434, error in (no error)=w428) -> (error out=w446:errorcluster)
        n174 = case shown="True" w443 {
          tunnel: w446 -> [w457 w461]
          tunnel: [w457 w460] -> w444
          tunnel: [w456 w459] -> w445
          tunnel: w440 -> [w456 w458]
          frame False {
          }
          frame True {
            n175 = property class="VI"(reference=w458, error in=w461) -> (reference out=w463:refnum<vi>, error out=w462:errorcluster, "Front Panel.Open"=w464:bool)
            n176 = case shown="True" w464 {
              tunnel: [w466 w470] -> w460
              tunnel: w462 -> [w466 w469]
              tunnel: w463 -> [w465 w468]
              tunnel: [w465 w467] -> w459
              frame False {
              }
              frame True {
                n177 = invoke class="VI" method="FP.Close"(reference=w468, error in=w469) -> (reference out=w467:refnum<vi>, error out=w470:errorcluster)  [unwired: 1 in, 1 out]
              }
            }
          }
        }
        n178 = Close Reference(reference=w445, error in (no error)=w444) -> (error out=w435:errorcluster)
      }
      frame "SEND MSG" {
        n179 = call-dynamic "Send Message.vi"("reference in"=w474, "error in (no error)"=w473, "Message (\"\" closes the window)"=w471) -> ("error out"=w472:errorcluster)  [unwired: 15 in, 1 out]
      }
      frame "CLOSE MSG" {
        n180 = call-dynamic "Send Message.vi"("reference in"=w478, "error in (no error)"=w479, "Message (\"\" closes the window)"="Close" ("Message")) -> ("error out"=w477:errorcluster)  [unwired: 15 in, 1 out]
      }
      frame "---- Miscelleneous ----" {
      }
      frame "unknown", Default {
        n181 = Concatenate Strings("The following state is unrecognized?\n", w485) -> (w484:string)
        n182 = One Button Dialog(message=w484) -> ()  [unwired: 1 in, 1 out]
      }
      frame "Error" {
        n183 = call <vilib>:"General Error Handler.vi"("error in (no error)"=w488) -> ()  [unwired: 10 in, 5 out]
      }
      frame "Next" {
        # "This is an empty case used so the queue does NOT stop if there is an empty string between two valid states!"
      }
      frame "Quit" {
        # "WARNING!, If the state machine crash, then it will also \"Quit\"??"
        # "This is the case used to simply exit when this GUI is used as a SubVI!"
        n184 = call-dynamic "Destroy.vi"("reference in"=w495, "error in (no error)"=w494) -> ("error out"=w493:errorcluster)  [unwired: 16 in, 1 out]
      }
    }
    "State Index" <- w18
  }
  "error out" <- w2
